vi "~sequence.vi"(6 "i":i32, 10 "Sequence":T4[](array[typedef])) -> (0 "Command":string, 1 "Attenuation dB":dbl, 2 "Phase Shift deg":dbl, 3 "NewSetup":T1, 4 "Sequence is done":bool)   [LabVIEW 2017]
uses:
  Classes/Sequence/SequenceSubvis/TestStep.ctl
  Classes/Sequence/SequenceSubvis/RF Direction.ctl
  Classes/Sequence/SequenceSubvis/PolarizationSelect.ctl
  Classes/Sequence/SequenceSubvis/PatchNewTestStep.ctl
panel:
  out "Test":T4
  # "This oject has members:\n- init\n- sequence\n- reset ?"
  # "NewStep\nNextPhaseShift\nNextAtten\nSequenceComplete"
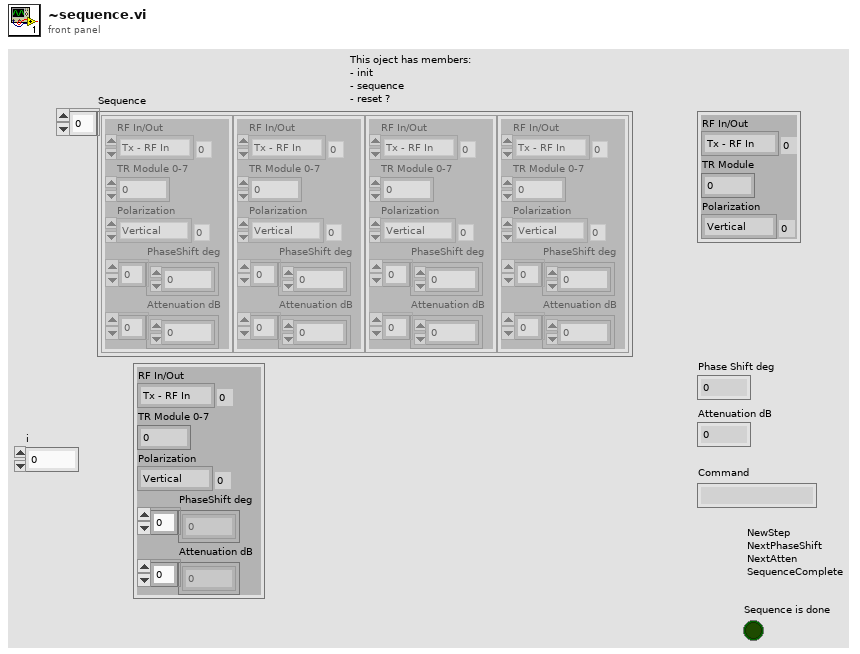
[diagram p1: front panel]
types:
  T1 = typedef "PatchNewTestStep.ctl" = cluster{"RF In/Out":T2, "TR Module":i32, "Polarization":T3}
  T2 = typedef "RF Direction.ctl" = enum16{"Tx - RF In", "Rx - RF Out"}
  T3 = typedef "PolarizationSelect.ctl" = enum16{"Vertical", "Horizontal"}
  T4 = typedef "TestStep.ctl" = cluster{"RF In/Out":T2, "TR Module 0-7":i32, "Polarization":T3, "PhaseShift deg":dbl[], "Attenuation dB":dbl[]}
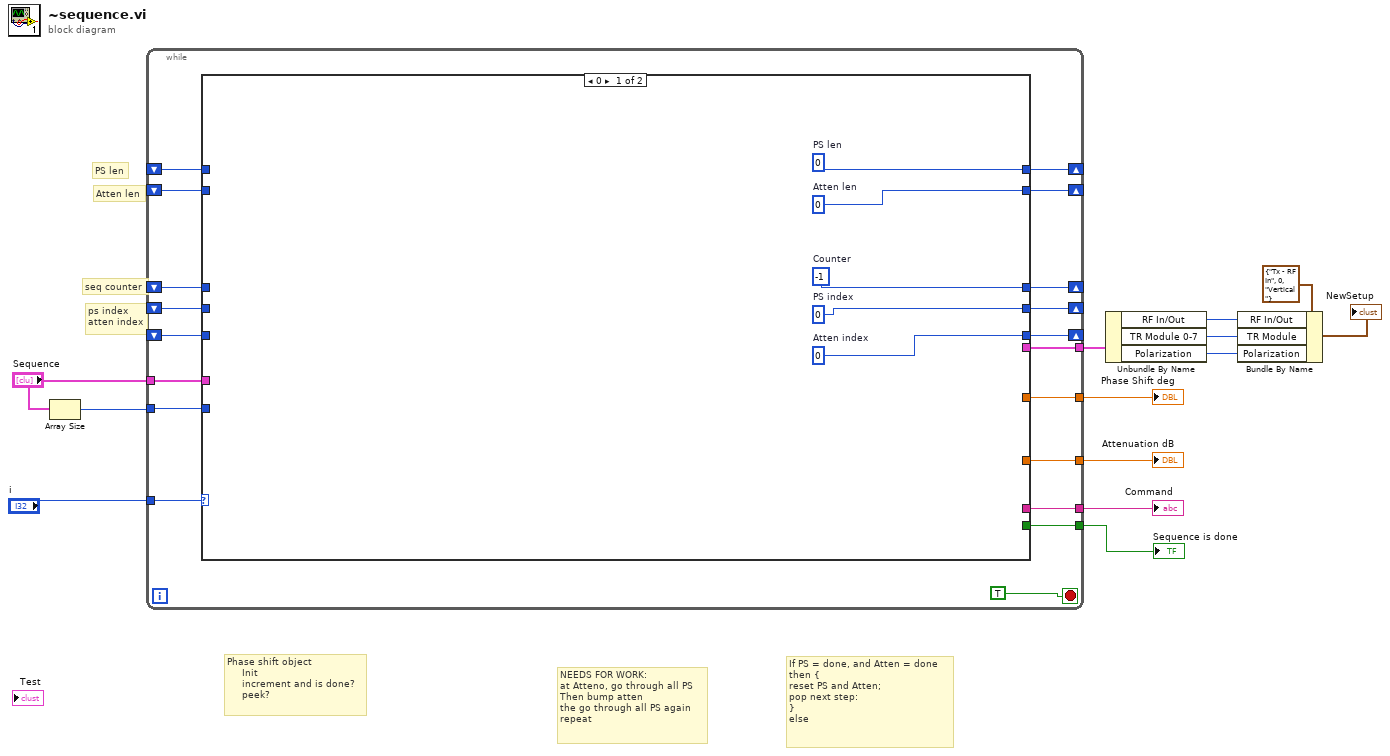
[diagram p0: block diagram]
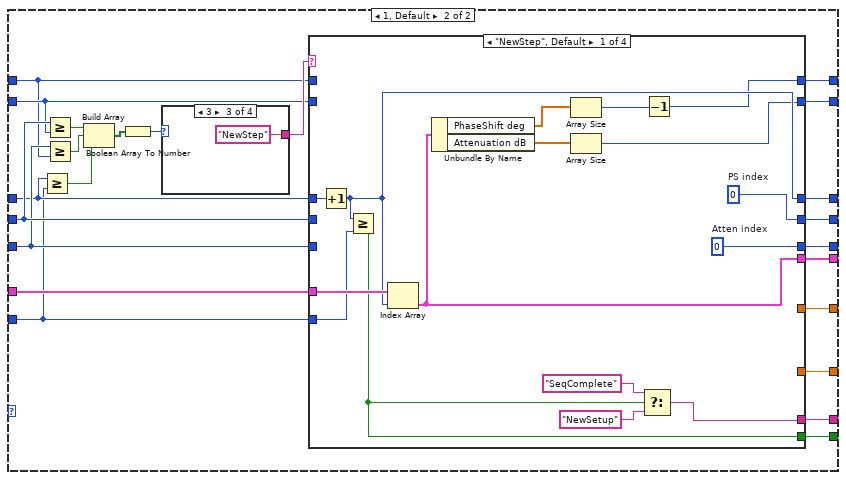
[diagram p2: hidden frame]
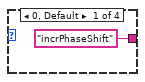
[diagram p3: hidden frame]
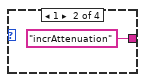
[diagram p4: hidden frame]
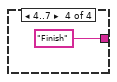
[diagram p5: hidden frame]
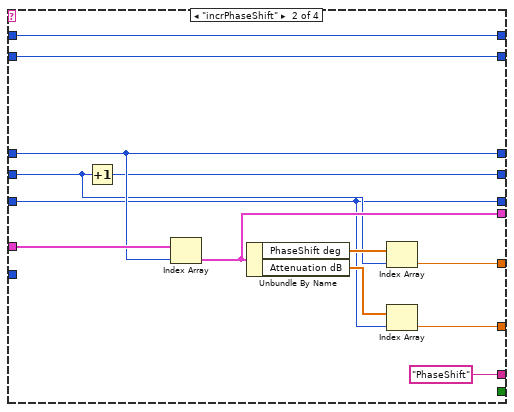
[diagram p6: hidden frame]
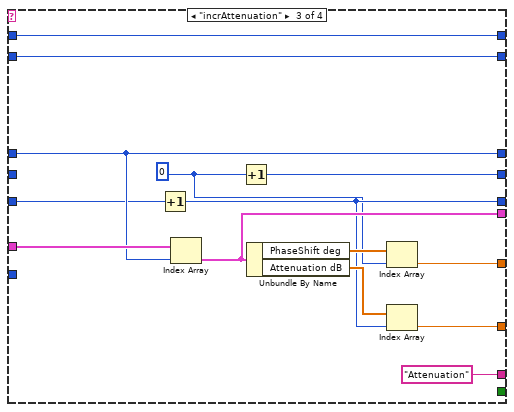
[diagram p7: hidden frame]
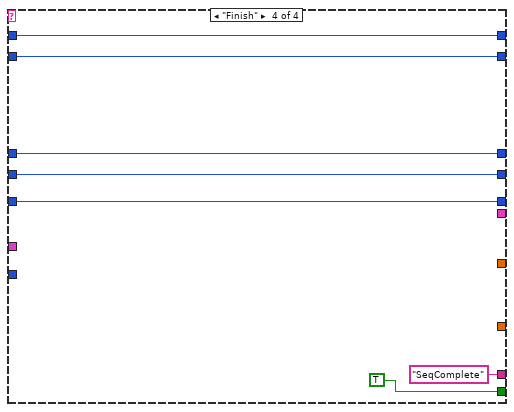
[diagram p8: hidden frame]
diagram:
  # "ps index\natten index"
  # "seq counter"
  # "Atten len"
  # "PS len"
  # "NEEDS FOR WORK:\nat Atteno, go through all PS\nThen bump atten\nthe go through all PS again\nrepeat"
  # "If PS = done, and Atten = done\nthen {\nreset PS and Atten;\npop next step:\n}\nelse"
  # "Phase shift object\n     Init\n     increment and is done?\n     peek?"
  n1 = Array Size(array="Sequence") -> (size(s)=w7:i32)
  n2 = while {
    shift-right: [w30] -> _
    shift-left: _ -> [w17]
    tunnel: "Sequence" -> [w29]
    shift-right: [w32] -> _
    shift-left: _ -> [w23]
    shift-right: [w31] -> _
    shift-left: _ -> [w22]
    shift-right: [w28] -> _
    shift-left: _ -> [w21]
    shift-right: [w27] -> _
    shift-left: _ -> [w20]
    tunnel: [w25] -> w6
    tunnel: [w24] -> w13
    tunnel: [w19] -> w12
    tunnel: [w18] -> w11
    tunnel: w7 -> [w16]
    tunnel: "i" -> [w15]
    tunnel: [w14] -> w8
    stop <- TRUE stop-if-true
    n3 = case shown="0" w15 {
      tunnel: [w34 w60] -> w32
      tunnel: [w33 w59] -> w31
      tunnel: [w35 w58] -> w30
      tunnel: w29 -> [_ w56]
      tunnel: [w36 w55] -> w28
      tunnel: [w37 w54] -> w27
      tunnel: [_ w53] -> w25
      tunnel: [_ w52] -> w24
      tunnel: w23 -> [_ w51]
      tunnel: w22 -> [_ w50]
      tunnel: w21 -> [_ w49]
      tunnel: w20 -> [_ w48]
      tunnel: [_ w43] -> w19
      tunnel: [_ w42] -> w18
      tunnel: w17 -> [_ w41]
      tunnel: w16 -> [_ w38]
      tunnel: [_ w39] -> w14
      frame 0 {
        w37 = 0  # PS len
        w36 = 0  # Atten len
        w33 = 0  # Atten index
        w34 = 0  # PS index
        w35 = -1  # Counter
      }
      frame 1, Default {
        n4 = Greater Or Equal?(x=w41, y=w38) -> (x >= y?=w40:bool)
        n5 = Greater Or Equal?(x=w51, y=w49) -> (x >= y?=w46:bool)
        n6 = Greater Or Equal?(x=w50, y=w48) -> (x >= y?=w47:bool)
        n7 = Build Array(w46, w47, w40) -> (w45:bool[])
        n8 = Boolean Array To Number(Boolean array=w45) -> (number=w44:u32)
        n9 = case shown="3" w44 {
          tunnel: ["incrPhaseShift" "incrAttenuation" "NewStep" "Finish"] -> w57
          frame 0, Default {
          }
          frame 1 {
          }
          frame 3 {
          }
          frame 4..7 {
          }
        }
        n10 = case shown="\"NewStep\", Default" w57 {
          tunnel: [w74 w87 w94 w113] -> w60
          tunnel: [w80 w83 w96 w114] -> w59
          tunnel: [w72 w92 w106 w112] -> w58
          tunnel: w41 -> [w78 w92 w106 w112]
          tunnel: w51 -> [_ w84 _ w113]
          tunnel: w50 -> [_ w83 w99 w114]
          tunnel: w56 -> [w79 w93 w107 _]
          tunnel: [w66 w89 w103 w110] -> w55
          tunnel: [w65 w88 w102 w111] -> w54
          tunnel: [w75 w91 w105 _] -> w53
          tunnel: [w68 "PhaseShift" ("Command") "Attenuation" ("Command") "SeqComplete" ("Command")] -> w52
          tunnel: w49 -> [_ w89 w103 w110]
          tunnel: w48 -> [_ w88 w102 w111]
          tunnel: [_ w82 w98 _] -> w43
          tunnel: [_ w81 w97 _] -> w42
          tunnel: [w67 _ _ TRUE] -> w39
          tunnel: w38 -> [w71 _ _ _]
          frame "NewStep", Default {
            w80 = 0  # Atten index
            w74 = 0  # PS index
            n11 = Increment(x=w78) -> (x+1=w72:i32)
            n12 = Greater Or Equal?(x=w72, y=w71) -> (x >= y?=w67:bool)
            n13 = Index Array(array=w79, index=w72) -> (element=w75:T4)
            n14 = Unbundle By Name(w75) -> ("PhaseShift deg"=w76:dbl[], "Attenuation dB"=w77:dbl[])
            n15 = Array Size(array=w76) -> (size(s)=w73:i32)
            n16 = Array Size(array=w77) -> (size(s)=w66:i32)
            n17 = Select(t="SeqComplete" ("Command"), s=w67, f="NewSetup" ("Command")) -> (s? t:f=w68:string)
            n18 = Decrement(x=w73) -> (x-1=w65:i32)
          }
          frame "incrPhaseShift" {
            n19 = Increment(x=w84) -> (x+1=w87:i32)
            n20 = Index Array(array=w93, index=w92) -> (element=w91:T4)
            n21 = Unbundle By Name(w91) -> ("PhaseShift deg"=w86:dbl[], "Attenuation dB"=w85:dbl[])
            n22 = Index Array(array=w86, index=w84) -> (element=w82:dbl)
            n23 = Index Array(array=w85, index=w83) -> (element=w81:dbl)
          }
          frame "incrAttenuation" {
            w95 = 0 ("PS index")
            n24 = Increment(x=w99) -> (x+1=w96:i32)
            n25 = Index Array(array=w107, index=w106) -> (element=w105:T4)
            n26 = Increment(x=w95) -> (x+1=w94:i32)
            n27 = Unbundle By Name(w105) -> ("PhaseShift deg"=w101:dbl[], "Attenuation dB"=w100:dbl[])
            n28 = Index Array(array=w101, index=w95) -> (element=w98:dbl)
            n29 = Index Array(array=w100, index=w96) -> (element=w97:dbl)
          }
          frame "Finish" {
          }
        }
      }
    }
  }
  "Command" <- w13
  "Sequence is done" <- w8
  "Phase Shift deg" <- w12
  "Attenuation dB" <- w11
  n30 = Unbundle By Name(w6) -> ("RF In/Out"=w5:T2, "TR Module 0-7"=w3:i32, "Polarization"=w2:T3)
  n31 = Bundle By Name(cluster=T1 {"RF In/Out"=enum."Tx - RF In", "TR Module"=0, "Polarization"=enum."Vertical"} ("NewSetup"), "RF In/Out"=w5, "TR Module"=w3, "Polarization"=w2) -> (→"NewSetup":T1)
